vi "run.exists.vi"(8 "error in":errorcluster, 10 "RunRid":string, 11 "Nominal Client in":refnum<class "Nominal Client.lvclass">) -> (0 "error out":errorcluster, 2 "Exists?":bool, 3 "Nominal Client out":refnum<class "Nominal Client.lvclass">)   [LabVIEW 2020, in "Nominal Client.lvclass"]
doc: "Checks if a Run exists"
uses:
  Nominal Client.lvclass
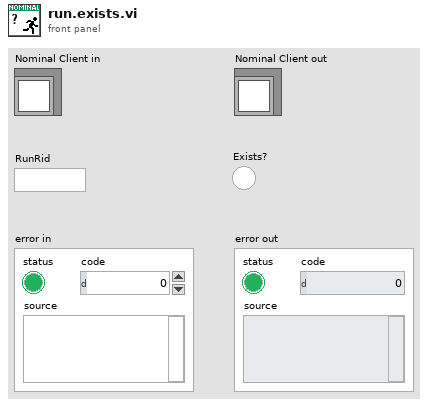
[diagram p1: front panel]
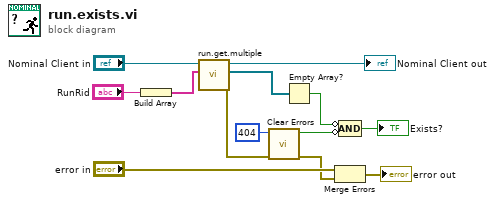
[diagram p0: block diagram]
diagram:
  n1 = Build Array("RunRid") -> (w2:string[])
  n2 = call "run.get.multiple.vi"("rid(s)"=w2, "Nominal Client in"="Nominal Client in") -> ("error out"=w10:errorcluster, "Runs"=w11:refnum<class "Run.lvclass">[], "Nominal Client out"=→"Nominal Client out":refnum<class "Nominal Client.lvclass">)  [unwired: 6 in, 1 out]
  n3 = call <vilib>:"Clear Errors.vi"("error in (no error)"=w10, "specific error code to clear (0: all)"=404) -> ("error out"=w7:errorcluster, "specific error cleared?"=w4:bool)  [unwired: 4 in]
  n4 = Empty Array?(array=w11) -> (empty?=w5:bool)
  n5 = Merge Errors("error in", w7) -> (→"error out":errorcluster)
  n6 = Compound Arithmetic op=AND(invert w5, invert w4) -> (→"Exists?":bool)
